vi "Init.vi"(8 "error in (no error)":errorcluster, 11 "User Data":T1) -> (0 "error out":errorcluster, 3 "SOL User out":refnum<class "SOL User.lvclass">)   [LabVIEW 2020, in "Summer of LabVIEW.lvlib" / "SOL User.lvclass"]
uses:
  SOL User.lvclass
  User Data.ctl
  SOL User.lvclass/SOL User.ctl
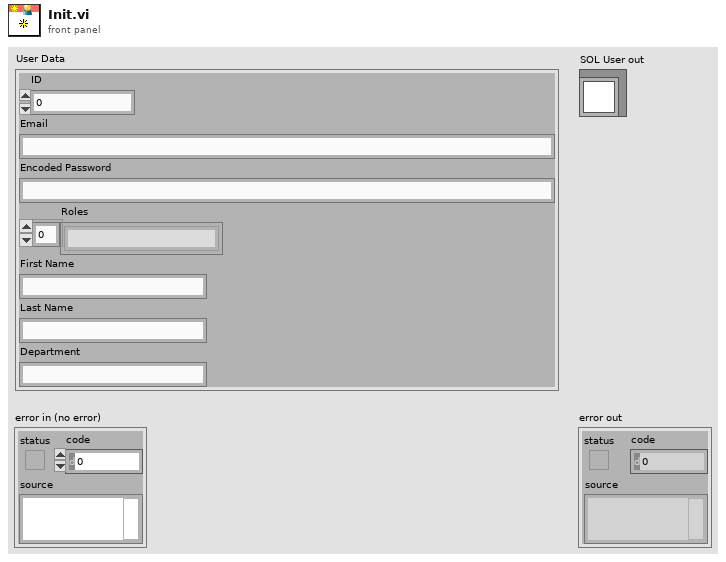
[diagram p1: front panel]
types:
  T1 = typedef "Summer of LabVIEW.lvlib/SOL User.lvclass/User Data.ctl" = cluster{"ID":i64, "Email":string, "Encoded Password":string, "Roles":string[], "First Name":string, "Last Name":string, "Department":string}
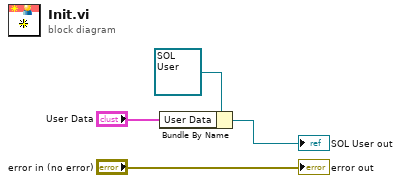
[diagram p0: block diagram]
diagram:
  n1 = Bundle By Name(cluster=refnum<class "SOL User.lvclass"> refnum ("SOL User out"), "User Data"="User Data") -> (→"SOL User out":refnum<class "SOL User.lvclass">)
  "error out" <- "error in (no error)"
